vi "task_2_b.vi"(0 "data":i32, 5 "Stop":bool, 7 "Operation":enum16{"get_value", "set_value", "Initialize"}(ring), 11 "error constant":errorcluster) -> (4 "data 2":i32, 6 "Stop 2":bool, 15 "error IO":errorcluster)   [LabVIEW 2023]
doc: "Store the data and stop values"
uses:
  task_2_b_op.ctl
  <vilib>/Utility/error.llb/DialogType.ctl
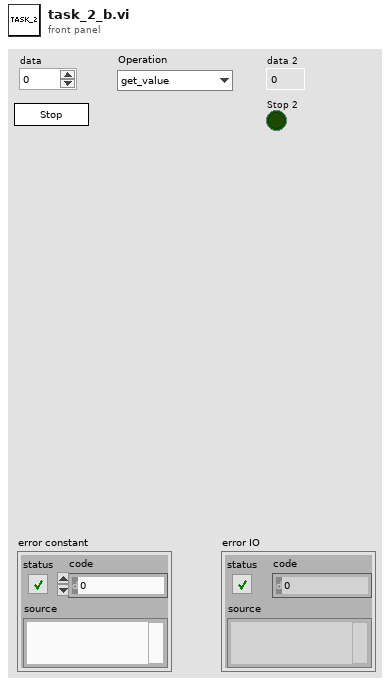
[diagram p1: front panel]
types:
  T1 = typedef "task_2_b_op.ctl" = cluster{"data":i32, "Stop":bool}
  T2 = typedef "DialogType.ctl" = u16
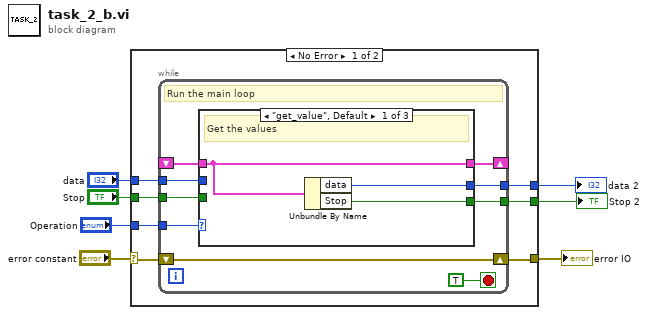
[diagram p0: block diagram]
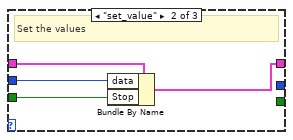
[diagram p2: hidden frame]
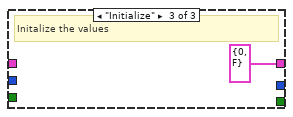
[diagram p3: hidden frame]
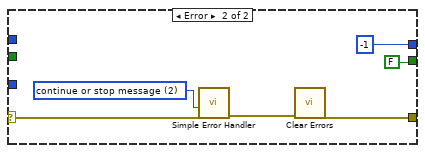
[diagram p4: hidden frame]
diagram:
  n1 = case shown="No Error" "error constant" {
    selector: "error constant" -> [w13 w37]
    tunnel: [w14 w34] -> w6
    tunnel: "Operation" -> [w12 _]
    tunnel: "Stop" -> [w11 _]
    tunnel: "data" -> [w10 _]
    tunnel: [w9 FALSE ("Stop")] -> w2
    tunnel: [w8 -1 ("data")] -> w1
    frame No Error {
      n2 = while {
        shift-right: [w20] -> _
        shift-left: _ -> [w19]
        tunnel: w12 -> [w21]
        tunnel: w11 -> [w18]
        tunnel: w10 -> [w17]
        tunnel: [w16] -> w9
        tunnel: [w15] -> w8
        shift-right: [w22] -> w14
        shift-left: w13 -> [w22]
        stop <- TRUE stop-if-true
        # "Run the main loop"
        n3 = case shown="\"get_value\", Default" w21 {
          tunnel: [w26 w29 T1 {"data"=0, "Stop"=FALSE}] -> w20
          tunnel: w19 -> [w26 w30 _]
          tunnel: w18 -> [_ w28 _]
          tunnel: w17 -> [_ w27 _]
          tunnel: [w25 _ _] -> w16
          tunnel: [w24 _ _] -> w15
          frame "get_value", Default {
            # "Get the values"
            n4 = Unbundle By Name(w26) -> ("data"=w24:i32, "Stop"=w25:bool)
          }
          frame "set_value" {
            # "Set the values"
            n5 = Bundle By Name(cluster=w30, "data"=w27, "Stop"=w28) -> (w29:T1)
          }
          frame "Initialize" {
            # "Initalize the values"
          }
        }
      }
    }
    frame Error {
      w35 = T2 2 items=["no dialog", "OK message", "continue or stop message", "OK message + warnings", "continue/stop + warnings"] ("type of dialog (OK msg:1)")
      n6 = call <vilib>:"Simple Error Handler.vi"("type of dialog (OK msg:1)"=w35, "error in (no error)"=w37) -> ("error out"=w36:errorcluster)  [unwired: 3 in, 4 out]
      n7 = call <vilib>:"Clear Errors.vi"("error in (no error)"=w36) -> ("error out"=w34:errorcluster)  [unwired: 5 in, 1 out]
    }
  }
  "error IO" <- w6
  "data 2" <- w1
  "Stop 2" <- w2
